vi "ANC300_Mode.vi"(0 "ANC300 Communication Port In":refnum<visa-resource-name>, 1 "connection ID in":refnum<k5>, 2 "Axis":u8(ring)=1 items=["1"=1, "2"=2, "3"=3, "4"=4, "5"=5, "6"=0], 3 "axis mode in":string(combo)="gnd", 5 "error in":T1, 6 "set / get":bool=TRUE, 7 "Time to wait [ms]":u32=200) -> (12 "command string":string, 13 "data out":string, 14 "ANC300 Communication Port Out":refnum<visa-resource-name>, 15 "connection ID out":refnum<k5>, 17 "axis mode out":string(combo)="gnd", 18 "transfer ok":bool, 19 "error out":T1)   [LabVIEW 2022 SP3]
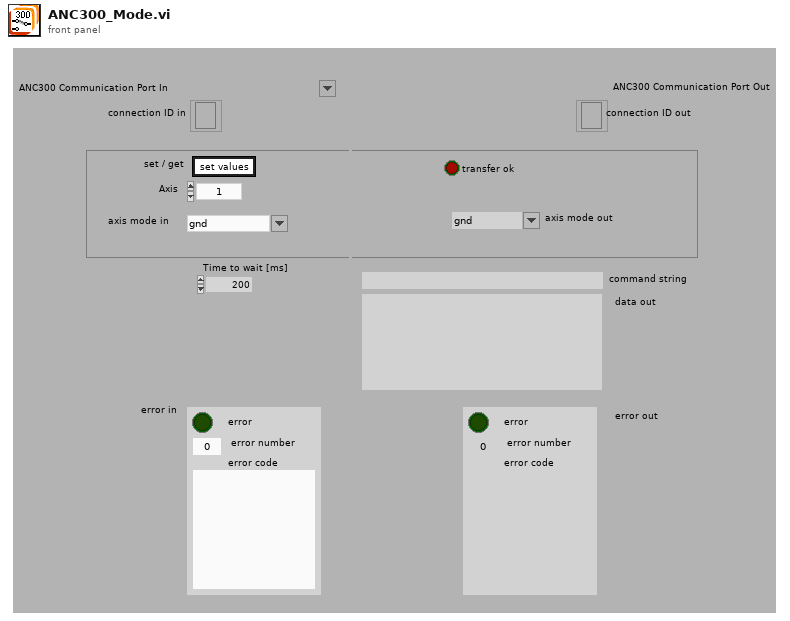
[diagram p1: front panel]
types:
  T1 = cluster{"error ":bool, "error number":i32, "error code":string}
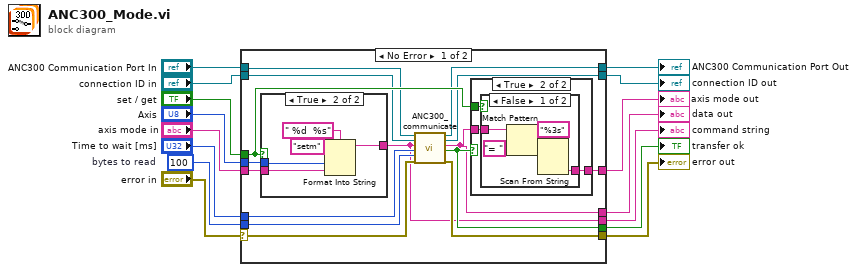
[diagram p0: block diagram]
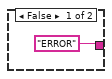
[diagram p2: hidden frame]
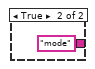
[diagram p3: hidden frame]
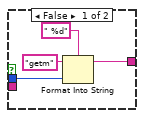
[diagram p4: hidden frame]
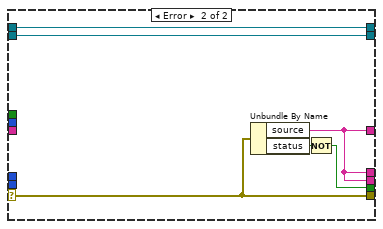
[diagram p5: hidden frame]
diagram:
  w10 = 100  # bytes to read
  n1 = case shown="No Error" "error in" {
    selector: "error in" -> [w19 w53]
    tunnel: "axis mode in" -> [w30 _]
    tunnel: "Axis" -> [w29 _]
    tunnel: "set / get" -> [w28 _]
    tunnel: "ANC300 Communication Port In" -> [w27 w55]
    tunnel: "connection ID in" -> [w26 w54]
    tunnel: "Time to wait [ms]" -> [w25 _]
    tunnel: w10 -> [w24 _]
    tunnel: [w23 w50] -> w1
    tunnel: [w22 w53] -> w4
    tunnel: [w21 w55] -> w8
    tunnel: [w20 w54] -> w7
    tunnel: [w18 w51] -> w3
    tunnel: [w17 w50] -> w6
    tunnel: [w16 w50] -> w5
    frame No Error {
      n2 = case shown="True" w28 {
        tunnel: w29 -> [w41 w46]
        tunnel: w30 -> [_ w45]
        tunnel: [w43 w48] -> w17
        frame False {
          n3 = Format Into String(format string=" %d", initial string="getm", w41) -> (resulting string=w43:string)  [unwired: 1 in, 1 out]
        }
        frame True {
          n4 = Format Into String(format string=" %d  %s", initial string="setm", w46, w45) -> (resulting string=w48:string)  [unwired: 1 in, 1 out]
        }
      }
      n5 = call "ANC300_communicate.vi"("ANC300 Communication Port In"=w27, "connection ID in"=w26, "commando string"=w17, "Time to wait [ms]"=w25, "bytes to read"=w24, "error in"=w19) -> ("ANC300 Communication Port Out"=w21:refnum<visa-resource-name>, "connection ID out"=w20:refnum<k5>, "read data"=w16:string, "transfer ok"=w18:bool, "error out"=w22:T1)  [unwired: 9 in]
      n6 = case shown="True" w18 {
        tunnel: ["ERROR" w34] -> w23
        tunnel: w16 -> [_ w33]
        tunnel: w28 -> [_ w32]
        frame False {
        }
        frame True {
          n7 = case shown="False" w32 {
            tunnel: w33 -> [w37 _]
            tunnel: [w35 "mode" ("data out")] -> w34
            frame False {
              n8 = Match Pattern(string=w37, regular expression="= ") -> (after substring=w39:string)  [unwired: 1 in, 3 out]
              n9 = Scan From String(format string="%3s", input string=w39) -> (output 1=w35:string)  [unwired: 3 in, 3 out]
            }
            frame True {
            }
          }
        }
      }
    }
    frame Error {
      n10 = Unbundle By Name(w53) -> ("source"=w50:string, "status"=w52:bool)
      n11 = Not(x=w52) -> (.not. x?=w51:bool)
    }
  }
  "data out" <- w5
  "connection ID out" <- w7
  "error out" <- w4
  "command string" <- w6
  "transfer ok" <- w3
  "ANC300 Communication Port Out" <- w8
  "axis mode out" <- w1
